vi "getDeviceCode.vi"(4 "handle":i32, 5 "错误输入（无错误）":errorcluster) -> (0 "return":i32, 1 "错误输出":errorcluster)   [LabVIEW 2013, in "EM_CVx.lvlib"]
uses:
  EM_CVx.lvlib
  library/moverLibrary_x86.dll
  library/moverLibrary_x64.dll
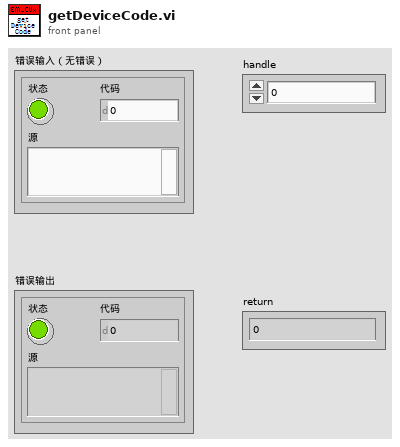
[diagram p1: front panel]
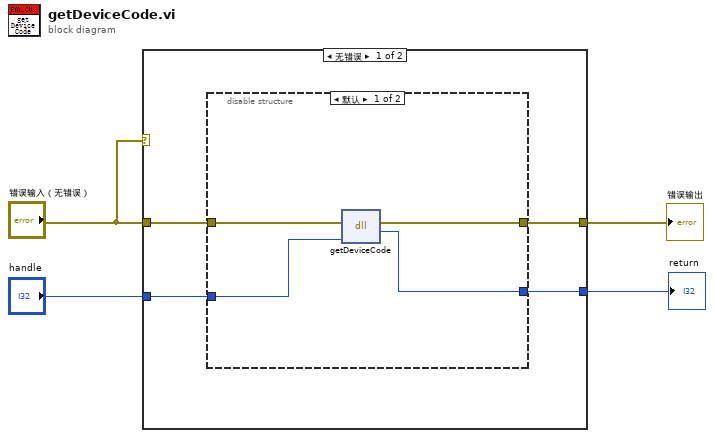
[diagram p0: block diagram]
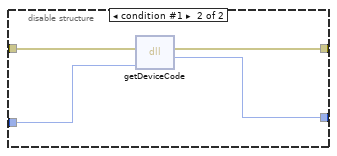
[diagram p2: hidden frame]
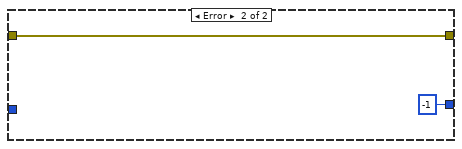
[diagram p3: hidden frame]
diagram:
  n1 = case shown="无错误" "错误输入（无错误）" {
    tunnel: "错误输入（无错误）" -> [w8 w18]
    tunnel: "handle" -> [w7 _]
    tunnel: [w6 w18] -> w3
    tunnel: [w5 -1 ("state")] -> w2
    frame No Error {
      n2 = disable-structure shown="默认" {
        disable-tunnel: w8 -> [w12 w16]
        disable-tunnel: w7 -> [w11 w14]
        disable-tunnel: [w10 w15] -> w6
        disable-tunnel: [w9 w13] -> w5
        frame condition #0 (active) {
          n3 = dll-call lib="E:/5-mover/4-labView/EM_CVx_2013/library/moverLibrary_x86.dll" fn="getDeviceCode"(error in=w12, "handle"=w11) -> (error out=w10:errorcluster, "return"=w9:i32)  [unwired: 3 in, 1 out]
        }
        frame condition #1 {
          n4 = dll-call lib="E:/5-mover/4-labView/EM_CVx_2013/library/moverLibrary_x64.dll" fn="getDeviceCode"(error in=w16, "handle"=w14) -> (error out=w15:errorcluster, "return"=w13:i32)  [unwired: 3 in, 1 out]
        }
      }
    }
    frame Error {
    }
  }
  "错误输出" <- w3
  "return" <- w2
